vi "LogTX.vi"(8 "error in (no error)":errorcluster, 11 "Stream in":refnum<class "Stream.lvclass">) -> (0 "error out":errorcluster, 3 "Stream out":refnum<class "Stream.lvclass">)   [LabVIEW 2018, in "Stream.lvclass"]
uses:
  Stream.lvclass
  Stream.lvclass/Stream.ctl
  Log/Log.lvclass
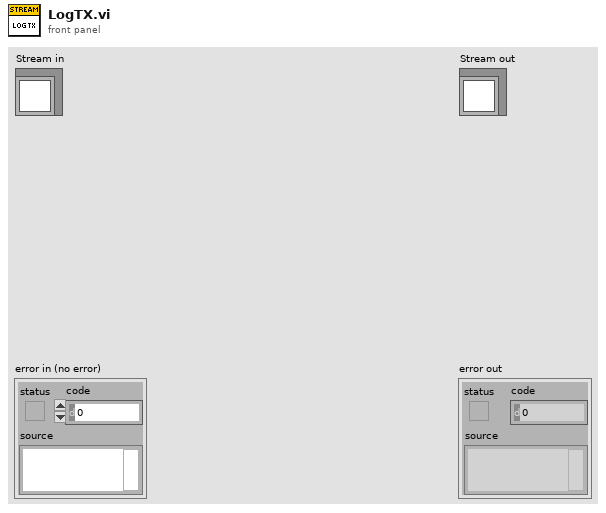
[diagram p1: front panel]
types:
  T1 = enum16{"INFO ", "TRACE", "DEBUG", "WARN ", "ERROR", "FATAL", "OTHER"}
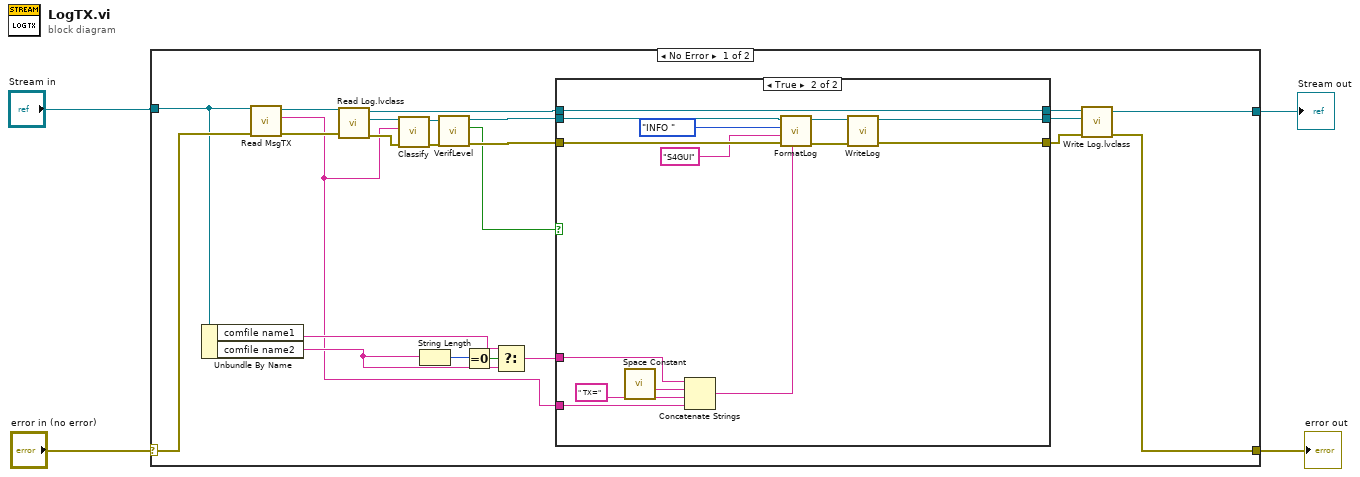
[diagram p0: block diagram]
diagram:
  n1 = case shown="No Error" "error in (no error)" {
    selector: "error in (no error)" -> [w27 w46]
    tunnel: [w24 w46] -> w1
    tunnel: [w23 w45] -> w2
    tunnel: "Stream in" -> [w26 w45]
    frame No Error {
      n2 = Unbundle By Name(w26) -> ("comfile name1"=w14:string, "comfile name2"=w15:string)
      n3 = call-dynamic "Read MsgTX.vi"("error in (no error)"=w27, "Comm in"=w26) -> ("error out"=w22:errorcluster, "MsgTX"=w6:string, "Comm out"=w25:refnum<class "Stream.lvclass">)  [unwired: 7 in]
      n4 = call-dynamic "Read Log.lvclass.vi"("error in (no error)"=w22, "Comm in"=w25) -> ("error out"=w19:errorcluster, "Log.lvclass"=w21:refnum<class "Log.lvclass">, "Comm out"=w13:refnum<class "Stream.lvclass">)  [unwired: 7 in]
      n5 = call-dynamic "Classify.vi"("error in (no error)"=w19, "msg to Log"=w6, "Log in"=w21) -> ("error out"=w18:errorcluster, "Log out"=w20:refnum<class "Log.lvclass">)  [unwired: 7 in]
      n6 = String Length(string=w15) -> (length=w16:i32)
      n7 = call-dynamic "VerifLevel.vi"("error in (no error)"=w18, "Log in"=w20) -> ("error out"=w11:errorcluster, "logging"=w7:bool, "Log out"=w12:refnum<class "Log.lvclass">)  [unwired: 7 in]
      n8 = Equal To 0?(x=w16) -> (x = 0?=w17:bool)
      n9 = Select(t=w14, s=w17, f=w15) -> (s? t:f=w5:string)
      n10 = case shown="True" w7 {
        tunnel: w13 -> [w30 w41]
        tunnel: w11 -> [w29 w36]
        tunnel: w6 -> [_ w43]
        tunnel: [w29 w34] -> w8
        tunnel: [w30 w41] -> w10
        tunnel: w5 -> [_ w42]
        tunnel: w12 -> [w28 w38]
        tunnel: [w28 w39] -> w9
        frame False {
        }
        frame True {
          n11 = call <vilib>:"Space Constant.vi"() -> ("String"=w40:string)
          n12 = Concatenate Strings(w42, w40, " TX=" ("string"), w43) -> (w32:string)
          n13 = call-dynamic "FormatLog.vi"("log input"=w32, "error in (no error)"=w36, "System"="S4GUI", "Type"=T1."INFO ", "Log in"=w38) -> ("error out"=w35:errorcluster, "Log out"=w37:refnum<class "Log.lvclass">)  [unwired: 5 in]
          n14 = call-dynamic "WriteLog.vi"("error in (no error)"=w35, "Log in"=w37) -> ("error out"=w34:errorcluster, "Log out"=w39:refnum<class "Log.lvclass">)  [unwired: 8 in]
        }
      }
      n15 = call-dynamic "Write Log.lvclass.vi"("error in (no error)"=w8, "Log.lvclass"=w9, "Comm in"=w10) -> ("error out"=w24:errorcluster, "Comm out"=w23:refnum<class "Stream.lvclass">)  [unwired: 7 in]
    }
    frame Error {
    }
  }
  "error out" <- w1
  "Stream out" <- w2
